vi "Set object text.vi"(8 "error in (no error)":errorcluster, 9 "Text":string, 10 "Object name":string, 11 "Domino Laser module Class in":refnum<class "Domino Laser module Class.lvclass">) -> (0 "error out":errorcluster, 1 "real":errorcluster, 2 "Command Excuted succeddfully?":bool, 3 "Domino Laser module Class out":refnum<class "Domino Laser module Class.lvclass">)   [LabVIEW 2015, in "Domino LM.lvlib" / "Domino Laser module Class.lvclass"]
uses:
  CTRLS/Domino Laser module Class.lvclass
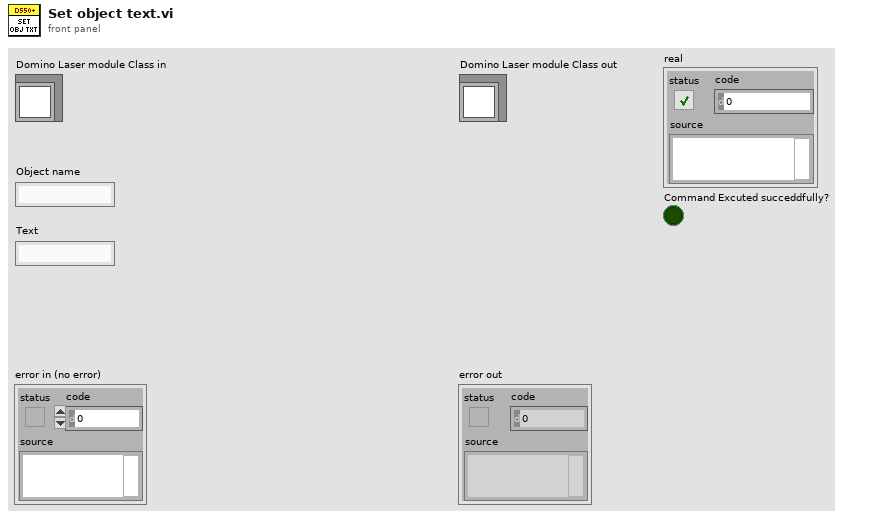
[diagram p1: front panel]
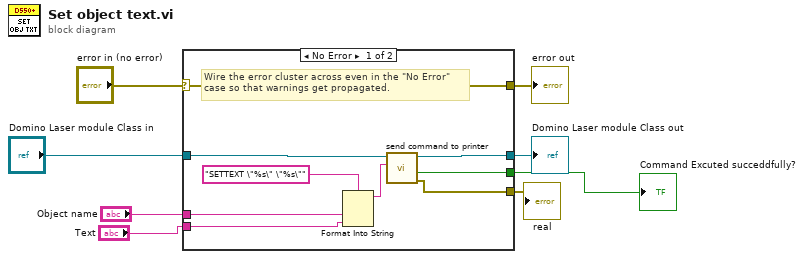
[diagram p0: block diagram]
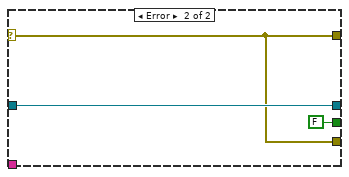
[diagram p2: hidden frame]
diagram:
  n1 = case shown="No Error" "error in (no error)" {
    selector: "error in (no error)" -> [w17 w19]
    tunnel: [w17 w19] -> w7
    tunnel: [w11 w20] -> w5
    tunnel: "Domino Laser module Class in" -> [w12 w20]
    tunnel: "Object name" -> [w15 _]
    tunnel: "Text" -> [w14 _]
    tunnel: [w10 w19] -> w2
    tunnel: [w9 FALSE ("Command Excuted succeddfully?")] -> w1
    frame No Error {
      # "Wire the error cluster across even in the \"No Error\"\ncase so that warnings get propagated."
      n2 = Format Into String(format string="SETTEXT \"%s\" \"%s\"", w15, w14) -> (resulting string=w13:string)  [unwired: 2 in, 1 out]
      n3 = call "send command to printer.vi"("command to be sent"=w13, "Domino Laser module Class in"=w12) -> ("error out"=w10:errorcluster, "Command Excuted succeddfully?"=w9:bool, "Domino Laser module Class out"=w11:refnum<class "Domino Laser module Class.lvclass">)  [unwired: 6 in, 1 out]
    }
    frame Error {
    }
  }
  "error out" <- w7
  "Domino Laser module Class out" <- w5
  "real" <- w2
  "Command Excuted succeddfully?" <- w1
